vi "PV ActiveLine - Pressure Unit.vi"(7 "W/R":bool, 8 "Fehler (Eingang)":errorcluster, 9 "Unit Set":i8(ring) items=["mbar / bar", "Torr", "Pascal", "Micron", "hPascal (default)", "Volt"], 11 "Referenz in":refnum<visa-resource-name>) -> (0 "Cluster (Ausgang)":errorcluster, 1 "Unit Get":i8(ring) items=["mbar / bar", "Torr", "Pascal", "Micron", "hPascal (default)", "Volt"], 3 "Referenz out":refnum<visa-resource-name>)   [LabVIEW 2013, in "PV ActiveLine.lvlib"]
doc: "Pressure unit \n\n0 –> mbar/bar\n1 –> Torr\n2 –> Pascal\n3 –> Micron\n4 –> hPascal (default)\n5 –> Volt"
uses:
  C:/Program Files (x86)/National Instruments/LabVIEW 2013/PV ActiveLine/PV ActiveLine.lvlib
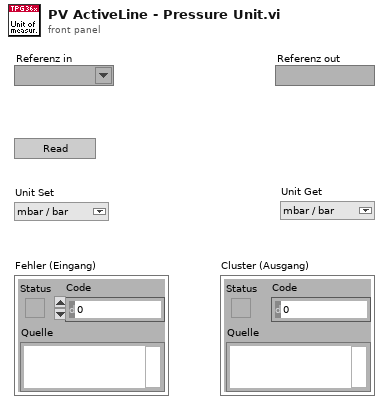
[diagram p1: front panel]
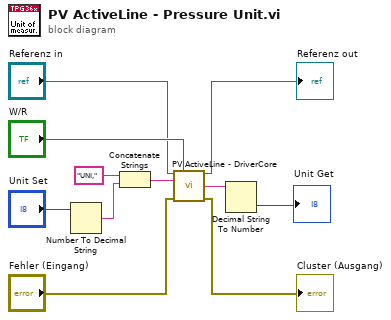
[diagram p0: block diagram]
diagram:
  n1 = Number To Decimal String(number="Unit Set") -> (decimal integer string=w7:string)  [unwired: 1 in]
  n2 = Concatenate Strings("UNI,", w7) -> (w5:string)
  n3 = call "PV ActiveLine - DriverCore.vi"("Referenz in"="Referenz in", "Write/Read"="W/R", "Command"=w5, "Fehler (Eingang)"="Fehler (Eingang)") -> ("Referenz out"=→"Referenz out":refnum<visa-resource-name>, "String Out"=w6:string, "Cluster (Ausgang)"=→"Cluster (Ausgang)":errorcluster)  [unwired: 9 in]
  n4 = Decimal String To Number(string=w6) -> (number=→"Unit Get":i32)  [unwired: 2 in, 1 out]
